vi "Client Begin Client Streaming Call.vi"(5 "Response Message Name":string, 6 "contextId":T1, 7 "Request Message Name":string, 8 "error in":errorcluster, 9 "timeout (ms)":i32=-1, 10 "Method Name":string, 11 "ClientID in":T1) -> (0 "error out":errorcluster, 2 "Call ID out":T1, 3 "ClientID out":T1)   [LabVIEW 2024, in "grpc-lvsupport.lvlib"]
uses:
  grpc-lvsupport.lvlib
  grpcId.ctl
  <vilib>/Utility/file.llb/Application Directory.vi
  <vilib>/Utility/error.llb/Error Cluster From Error Code.vi
  <resource>/labview_grpc_server.dll
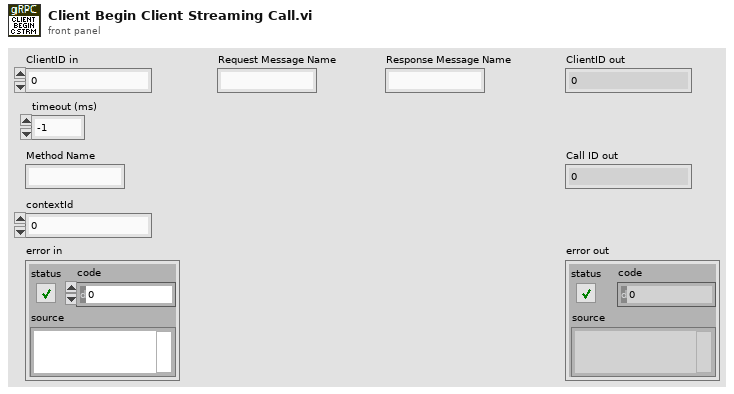
[diagram p1: front panel]
types:
  T1 = typedef "grpc-lvsupport.lvlib/grpcId.ctl" = u64
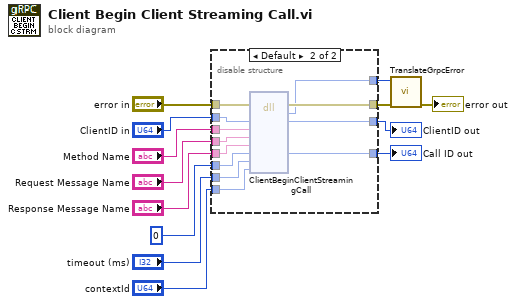
[diagram p0: block diagram]
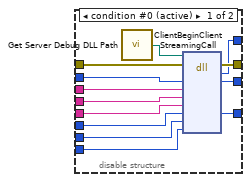
[diagram p2: hidden frame]
diagram:
  n1 = disable-structure shown="Default" {
    disable-tunnel: "error in" -> [w26 w38]
    disable-tunnel: [w25 w37] -> w12
    disable-tunnel: [w23 w36] -> w11
    disable-tunnel: "ClientID in" -> [w22 w35]
    disable-tunnel: "Response Message Name" -> [w21 w34]
    disable-tunnel: "Request Message Name" -> [w20 w33]
    disable-tunnel: "Method Name" -> [w19 w32]
    disable-tunnel: [w18 w31] -> w6
    disable-tunnel: [w17 w30] -> w4
    disable-tunnel: "timeout (ms)" -> [w16 w29]
    disable-tunnel: "contextId" -> [w15 w28]
    disable-tunnel: u64 0 ("callId") -> [w14 w27]
    frame condition #0 (active) {
      n2 = call "Get Server Debug DLL Path.vi"() -> ("DLL Path"=w24:path)
      n3 = dll-call lib="?" fn="ClientBeginClientStreamingCall"(path in=w24, error in=w26, "ClientId"=w22, "methodName"=w19, "requestMessageName"=w20, "responseMessageName"=w21, "callId"=w14, "timeoutMs"=w16, "contextId"=w15) -> (error out=w25:errorcluster, "return type"=w17:i32, "ClientId"=w18:u64, "callId"=w23:u64)  [unwired: 6 in, 1 out]
    }
    frame condition #1 {
      n4 = dll-call lib="C:/Program Files (x86)/National Instruments/LabVIEW 2024/resource/labview_grpc_server.*" fn="ClientBeginClientStreamingCall"(error in=w38, "ClientId"=w35, "methodName"=w32, "requestMessageName"=w33, "responseMessageName"=w34, "callId"=w27, "timeoutMs"=w29, "contextId"=w28) -> (error out=w37:errorcluster, "return type"=w30:i32, "ClientId"=w31:u64, "callId"=w36:u64)  [unwired: 7 in, 1 out]
    }
  }
  "ClientID out" <- w6
  "Call ID out" <- w11
  n5 = call "TranslateGrpcError.vi"("error in"=w12, "Error Code"=w4) -> ("error out"=→"error out":errorcluster)  [unwired: 9 in]
